vi "CommonVIs_SetVimProperties.vi"(8 "error in (no error)":errorcluster, 11 "VIRefIn":refnum<vi>) -> (0 "error out":errorcluster, 3 "VIRefOut":refnum<vi>)   [LabVIEW 2020]
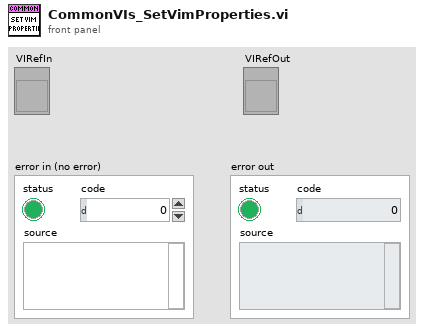
[diagram p1: front panel]
types:
  T1 = enum16{"Invalid Wire Rule", "Required", "Recommended", "Optional", "Dynamic Dispatch"}
  T2 = enum16{"Share clones between instances", "Preallocate clone for each instance"}
  T3 = typedef "LVRectTypeDef.ctl" = cluster{"Left":i16, "Top":i16, "Right":i16, "Bottom":i16}
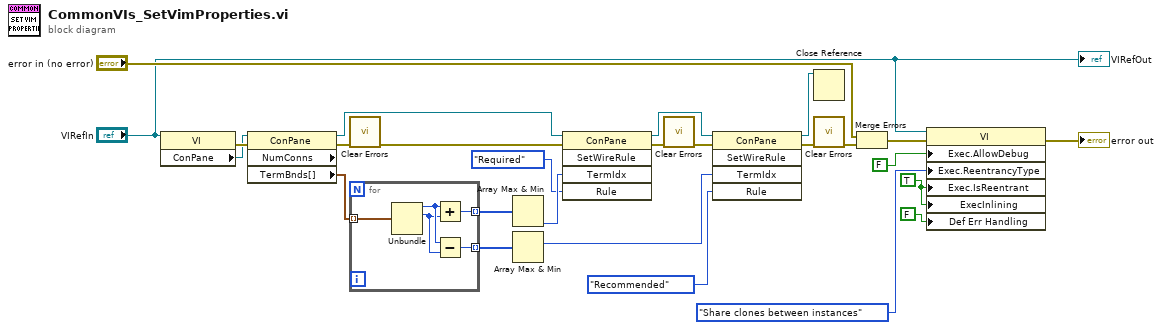
[diagram p0: block diagram]
diagram:
  w24 = TRUE ("Execution:Is Reentrant")
  n1 = property class="VI"(reference="VIRefIn") -> (error out=w21:errorcluster, "ConPane"=w15:refnum<vi>)  [unwired: 1 in, 1 out]
  n2 = property class="ConPane" props=["NumConns", "TermBnds[]"](reference=w15, error in=w21) -> (reference out=w16:refnum<vi>, error out=w17:errorcluster, "TermBnds[]"=w10:T3[])  [unwired: 1 out]
  n3 = call <vilib>:"Clear Errors.vi"("error in (no error)"=w17) -> ("error out"=w7:errorcluster)  [unwired: 5 in, 1 out]
  n4 = for {
    tunnel: w10 -> [w31] mode=indexing
    tunnel: [w30] -> w9 mode=indexing
    tunnel: [w27] -> w8 mode=indexing
    n5 = Unbundle(w31) -> ("Left"=w29:i16, "Top"=w28:i16)  [unwired: 2 out]
    n6 = Add(x=w29, y=w28) -> (x+y=w30:i16)
    n7 = Subtract(x=w29, y=w28) -> (x-y=w27:i16)
  }
  n8 = Array Max & Min(array=w9) -> (min index (indices)=w18:i32)  [unwired: 3 out]
  n9 = Array Max & Min(array=w8) -> (max index (indices)=w19:i32)  [unwired: 3 out]
  n10 = invoke class="ConPane" method="SetWireRule"(reference=w16, error in=w7, "TermIdx"=w18, "Rule"=T1."Required") -> (reference out=w13:refnum<vi>, error out=w14:errorcluster)  [unwired: 1 in, 3 out]
  n11 = call <vilib>:"Clear Errors.vi"("error in (no error)"=w14) -> ("error out"=w6:errorcluster)  [unwired: 5 in, 1 out]
  n12 = invoke class="ConPane" method="SetWireRule"(reference=w13, error in=w6, "TermIdx"=w19, "Rule"=T1."Recommended") -> (reference out=w20:refnum<vi>, error out=w5:errorcluster)  [unwired: 1 in, 3 out]
  n13 = Close Reference(reference=w20) -> ()  [unwired: 1 in, 1 out]
  n14 = call <vilib>:"Clear Errors.vi"("error in (no error)"=w5) -> ("error out"=w4:errorcluster)  [unwired: 5 in, 1 out]
  n15 = Merge Errors("error in (no error)", w4) -> (w2:errorcluster)
  n16 = property class="VI"(reference="VIRefIn", error in=w2, "Exec.AllowDebug"=FALSE ("Execution:Allow Debugging"), "Exec.ReentrancyType"=T2."Share clones between instances" ("Execution:Reentrancy Type"), "Exec.IsReentrant"=w24, "ExecInlining"=w24, "Def Err Handling"=FALSE ("Execution:Allow Debugging")) -> (error out=→"error out":errorcluster)  [unwired: 1 out]
  "VIRefOut" <- "VIRefIn"
